vi "ABC Find Close - Front.vi"(4 "UART":refnum<vi>, 5 "ComPort":refnum<visa-resource-name>, 6 "Data":refnum<vi>, 7 "DaqTask":refnum<k21>, 8 "ErrIn":errorcluster, 9 "#Step":i32, 10 "Dir":T1, 11 "DataIn":dbl[](array[numeric])=[0.0]) -> (0 "ErrOut":errorcluster, 1 "FrontClose":dbl, 3 "DataOut":dbl[](array[numeric]))   [LabVIEW 2020]
uses:
  <userlib>/Amira UART/Public/TypeDefs/AUART StepDir.ctl
  <vilib>/DAQmx/read.llb/DAQmx Read (Digital 1D Bool 1Chan 1Samp).vi
  <vilib>/DAQmx/miscellaneous.llb/DAQmx Fill In Error Info.vi
  <userlib>/Amira UART/Amira UART.lvclass
  <userlib>/KQD LabVIEW User/Serial/Serial.lvlib
panel:
  out "FrontSW":bool
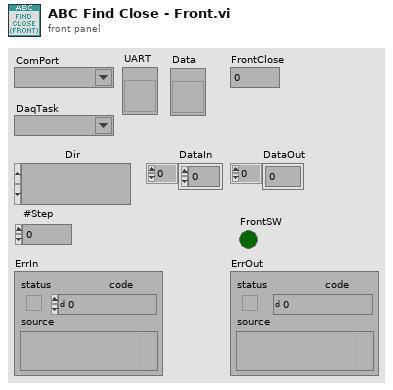
[diagram p1: front panel]
types:
  T1 = typedef "Amira UART.lvclass/AUART StepDir.ctl" = enum16{"", "compress", "decompress"}
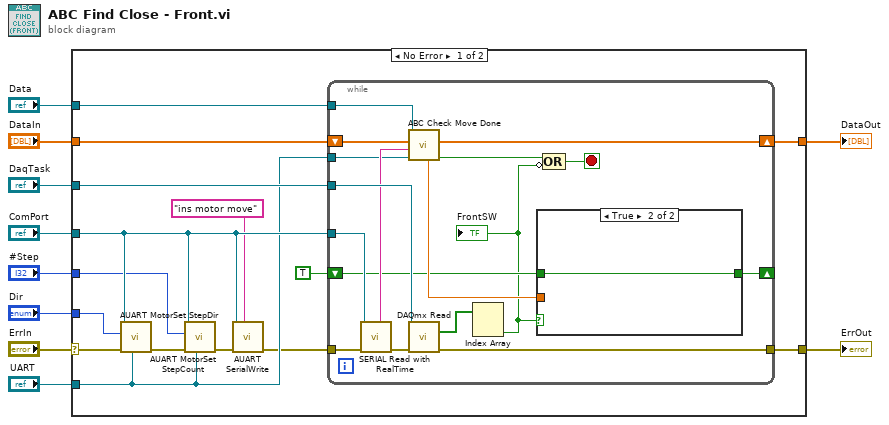
[diagram p0: block diagram]
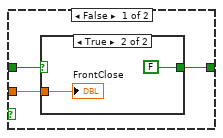
[diagram p2: hidden frame]
diagram:
  n1 = case shown="No Error" "ErrIn" {
    selector: "ErrIn" -> [w19 w50]
    tunnel: "UART" -> [w18 _]
    tunnel: "DaqTask" -> [w25 _]
    tunnel: [w24 w50] -> w8
    tunnel: "DataIn" -> [w23 w51]
    tunnel: [w22 w51] -> w6
    tunnel: "ComPort" -> [w20 _]
    tunnel: "Data" -> [w17 _]
    tunnel: "Dir" -> [w13 _]
    tunnel: "#Step" -> [w12 _]
    frame No Error {
      n2 = call <userlib>:"AUART MotorSet StepDir.vi"("UART"=w18, "ErrIn"=w19, "step_dir"=w13, "Port"=w20) -> ("ErrOut"=w21:errorcluster)  [unwired: 7 in]
      n3 = call <userlib>:"AUART MotorSet StepCount.vi"("UART"=w18, "ErrIn"=w21, "step_count"=w12, "Port"=w20) -> ("ErrOut"=w16:errorcluster)  [unwired: 7 in]
      n4 = call <userlib>:"AUART SerialWrite.vi"("Cmd"="ins motor move", "ErrIn"=w16, "Port"=w20) -> ("ErrOut"=w15:errorcluster)  [unwired: 7 in, 1 out]
      n5 = while {
        tunnel: w25 -> [w41]
        tunnel: w17 -> [w35]
        tunnel: w20 -> [w40]
        shift-right: [w32] -> w22
        shift-left: w23 -> [w36]
        tunnel: w15 -> [w39]
        tunnel: [w37] -> w24
        tunnel: w18 -> [w33]
        shift-right: [w27] -> _
        shift-left: TRUE -> [w28]
        stop <- w30 stop-if-true
        n6 = call <userlib>:"SERIAL Read with RealTime.vi"("ErrIn"=w39, "PortIn"=w40) -> ("ErrOut"=w38:errorcluster, "Response"=w34:string)  [unwired: 7 in, 1 out]
        n7 = call "ABC Check Move Done.vi"("UART"=w33, "Response"=w34, "DataIn"=w36, "Data"=w35) -> ("Done"=w29:bool, "DataOut"=w32:dbl[], "Position"=w31:dbl)  [unwired: 5 in]
        n8 = call-poly <vilib>:"DAQmx Read.vi"("task/channels in"=w41, "error in"=w38) -> ("data"=w42:bool[], "error out"=w37:errorcluster)  [unwired: 11 in, 1 out]
        n9 = Index Array(array=w42) -> (element #2=w26:bool)  [unwired: 2 in, 1 out]
        "FrontSW" <- w26
        n10 = case shown="True" w26 {
          tunnel: w31 -> [w45 _]
          tunnel: w28 -> [w44 w49]
          tunnel: [w43 w49] -> w27
          frame False {
            n11 = case shown="True" w44 {
              selector: w44 -> [w46 _]
              tunnel: w45 -> [_ w48]
              tunnel: [w46 FALSE] -> w43
              frame False {
              }
              frame True {
                "FrontClose" <- w48
              }
            }
          }
          frame True {
          }
        }
        n12 = Compound Arithmetic op=OR(w29, invert w26) -> (w30:bool)
      }
    }
    frame Error {
    }
  }
  "ErrOut" <- w8
  "DataOut" <- w6
